vi "If Else X.vi"(0 "denge degeri":dbl, 5 "Xk":dbl, 7 "X(k-1)":dbl=0.1, 9 "output x 1":dbl, 11 "output x 2":dbl, 12 "result output x":dbl) -> (4 "Output X(k-1)":dbl format="%.4p", 15 "Start X":bool)   [LabVIEW 2014]
uses:
  Sub_VI/show_sensitivity.vi
  Sub_VI/global get findinput.vi
panel:
  out "cycle":bool
  in  "GPIB In":refnum<visa-resource-name>="GPIB0::8::INSTR"
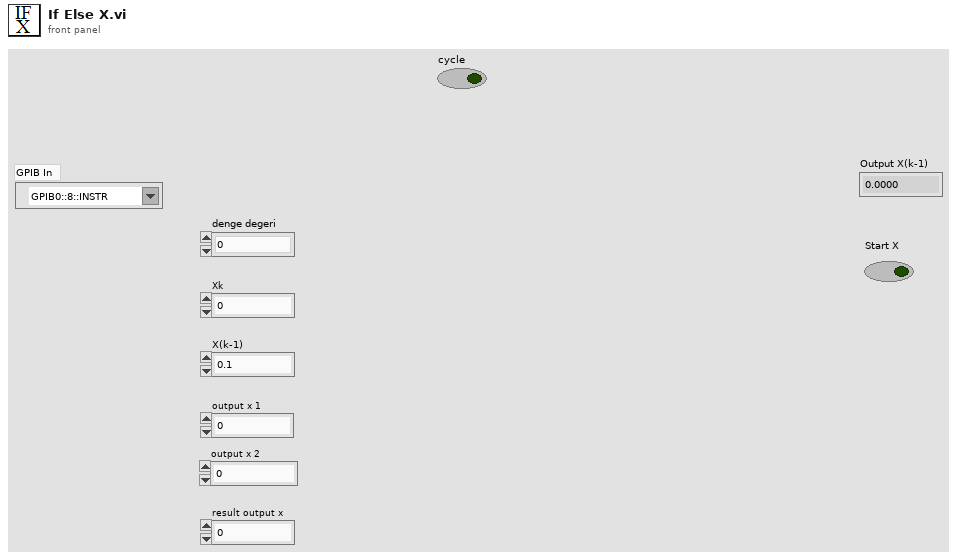
[diagram p1: front panel]
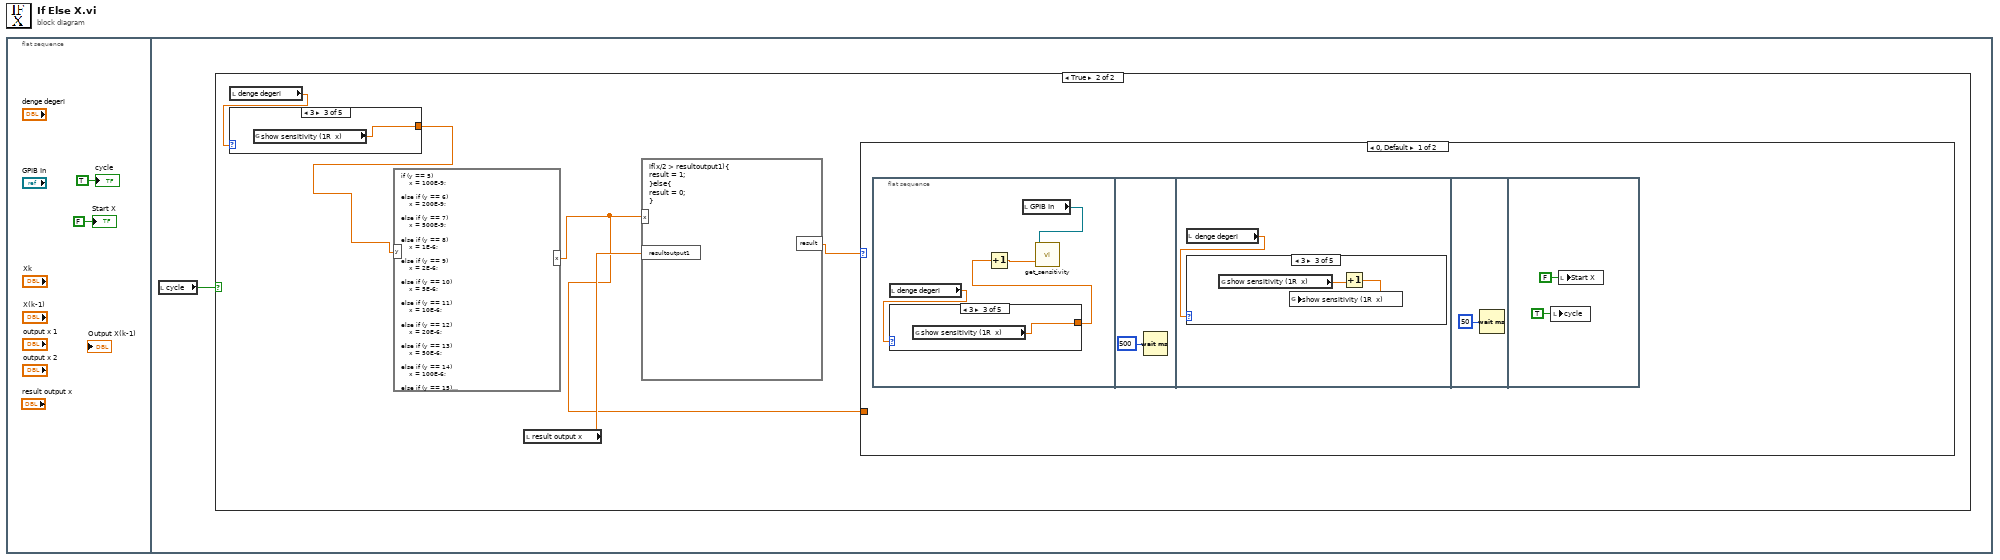
[diagram p0: block diagram]
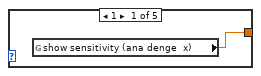
[diagram p3: hidden frame]
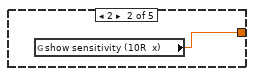
[diagram p4: hidden frame]
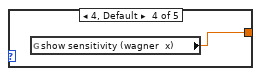
[diagram p5: hidden frame]
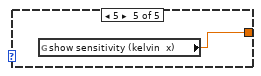
[diagram p6: hidden frame]
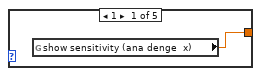
[diagram p7: hidden frame]
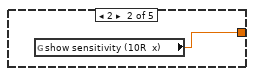
[diagram p8: hidden frame]
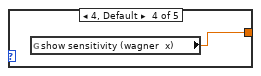
[diagram p9: hidden frame]
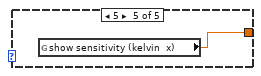
[diagram p10: hidden frame]
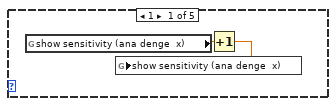
[diagram p11: hidden frame]
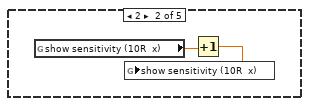
[diagram p12: hidden frame]
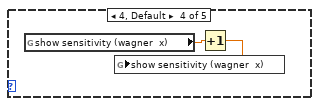
[diagram p13: hidden frame]
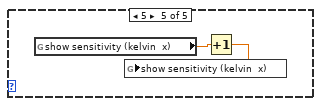
[diagram p14: hidden frame]
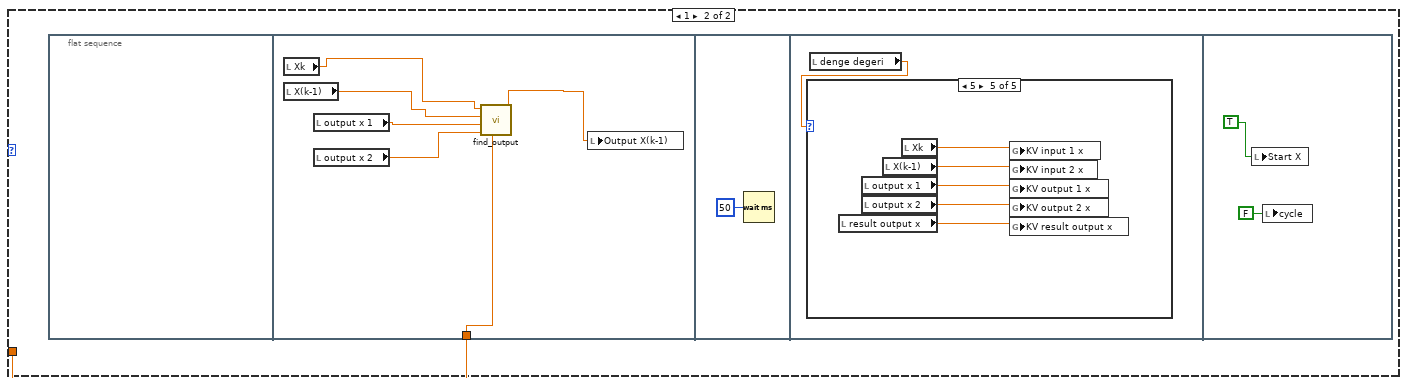
[diagram p15: hidden frame]
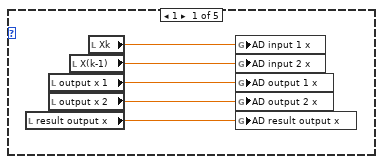
[diagram p16: hidden frame]
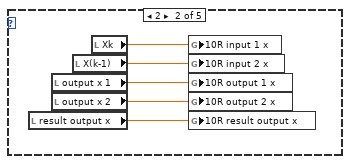
[diagram p17: hidden frame]
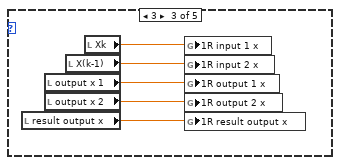
[diagram p18: hidden frame]
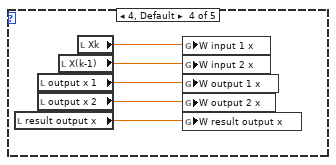
[diagram p19: hidden frame]
diagram:
  n1 = flat-sequence {
    frame #0 {
      "Start X" <- FALSE ("Start X")
      "cycle" <- TRUE ("Boolean")
    }
    frame #1 {
      n2 = local read "cycle"() -> (w3:bool)
      n3 = case shown="True" w3 {
        frame False {
        }
        frame True {
          n4 = local read "denge degeri"() -> (w5:dbl)
          n5 = case shown="3" w5 {
            tunnel: [w9 w10 w11 w12 w13] -> w4
            frame 1 {
              n6 = global read "show_sensitivity.vi" "show sensitivity (ana denge  x)"() -> (w9:dbl)
            }
            frame 2 {
              n7 = global read "show_sensitivity.vi" "show sensitivity (10R  x)"() -> (w10:dbl)
            }
            frame 3 {
              n8 = global read "show_sensitivity.vi" "show sensitivity (1R  x)"() -> (w11:dbl)
            }
            frame 4, Default {
              n9 = global read "show_sensitivity.vi" "show sensitivity (wagner  x)"() -> (w12:dbl)
            }
            frame 5 {
              n10 = global read "show_sensitivity.vi" "show sensitivity (kelvin  x)"() -> (w13:dbl)
            }
          }
          n11 = formula code="if (y == 5) \n    x = 100E-9;\n\nelse if (y == 6) \n    x = 200E-9;\n\nelse if (y == 7) \n    x = 500E-9;\n\nelse if (y == 8) \n    x = 1E-6;\n\nelse if (y == 9) \n    x = 2E-6;\n\nelse if (y == 10) \n    x = 5E-6;\n\nelse if (y == 11) \n    x = 10E-6;\n\nelse if (y == 12) \n    x = 20E-6;\n\nelse if (y == 13) \n    x = 50E-6;\n\nelse if (y == 14) \n    x = 100E-6;\n\nelse if (y == 15) \n    x = 200E-6;\n\nelse if (y == 16) \n    x = 500E-6;\n\nelse if (y == 17) \n    x = 1E-3;\n\nelse if (y == 18) \n    x = 2E-3;\n\nelse if (y == 19) \n    x = 5E-3;\n\nelse if (y == 20) \n    x = 10E-3;\n\nelse if (y == 21) \n    x = 20E-3;\n\nelse if (y == 22) \n    x = 50E-3;\n\nelse if (y == 23) \n    x = 100E-3;\n\nelse if (y == 24) \n    x = 200E-3;\n\nelse if (y == 25) \n    x = 500E-3;\n\nelse if (y == 26) \n    x = 1;\n\nelse \n    x = 1;"("y"=w4) -> ("x"=w6:dbl)
          n12 = local read "result output x"() -> (w8:dbl)
          n13 = formula code="if(x/2 > resultoutput1){\nresult = 1;\n}else{\nresult = 0;\n}"("x"=w6, "resultoutput1"=w8) -> ("result"=w7:dbl)
          n14 = case shown="0, Default" w7 {
            tunnel: w6 -> [_ w38]
            frame 0, Default {
              n15 = flat-sequence {
                frame #0 {
                  n16 = local read "denge degeri"() -> (w15:dbl)
                  n17 = case shown="3" w15 {
                    tunnel: [w18 w19 w20 w21 w22] -> w14
                    frame 1 {
                      n18 = global read "show_sensitivity.vi" "show sensitivity (ana denge  x)"() -> (w18:dbl)
                    }
                    frame 2 {
                      n19 = global read "show_sensitivity.vi" "show sensitivity (10R  x)"() -> (w19:dbl)
                    }
                    frame 3 {
                      n20 = global read "show_sensitivity.vi" "show sensitivity (1R  x)"() -> (w20:dbl)
                    }
                    frame 4, Default {
                      n21 = global read "show_sensitivity.vi" "show sensitivity (wagner  x)"() -> (w21:dbl)
                    }
                    frame 5 {
                      n22 = global read "show_sensitivity.vi" "show sensitivity (kelvin  x)"() -> (w22:dbl)
                    }
                  }
                  n23 = Increment(x=w14) -> (x+1=w16:dbl)
                  n24 = local read "GPIB In"() -> (w17:refnum<visa-resource-name>)
                  n25 = call "get_sensitivity.vi"("input 1"=w16, "SR850 GPIB In"=w17) -> ()  [unwired: 8 in, 2 out]
                }
                frame #1 {
                  n26 = Wait (ms)(milliseconds to wait=u32 500) -> ()  [unwired: 1 out]
                }
                frame #2 {
                  n27 = local read "denge degeri"() -> (w24:dbl)
                  n28 = case shown="3" w24 {
                    frame 1 {
                      n29 = global read "show_sensitivity.vi" "show sensitivity (ana denge  x)"() -> (w26:dbl)
                      n30 = Increment(x=w26) -> (x+1=w25:dbl)
                      n31 = global write "show_sensitivity.vi" "show sensitivity (ana denge  x)"(w25) -> ()
                    }
                    frame 2 {
                      n32 = global read "show_sensitivity.vi" "show sensitivity (10R  x)"() -> (w28:dbl)
                      n33 = Increment(x=w28) -> (x+1=w27:dbl)
                      n34 = global write "show_sensitivity.vi" "show sensitivity (10R  x)"(w27) -> ()
                    }
                    frame 3 {
                      n35 = global read "show_sensitivity.vi" "show sensitivity (1R  x)"() -> (w30:dbl)
                      n36 = Increment(x=w30) -> (x+1=w29:dbl)
                      n37 = global write "show_sensitivity.vi" "show sensitivity (1R  x)"(w29) -> ()
                    }
                    frame 4, Default {
                      n38 = global read "show_sensitivity.vi" "show sensitivity (wagner  x)"() -> (w32:dbl)
                      n39 = Increment(x=w32) -> (x+1=w31:dbl)
                      n40 = global write "show_sensitivity.vi" "show sensitivity (wagner  x)"(w31) -> ()
                    }
                    frame 5 {
                      n41 = global read "show_sensitivity.vi" "show sensitivity (kelvin  x)"() -> (w34:dbl)
                      n42 = Increment(x=w34) -> (x+1=w33:dbl)
                      n43 = global write "show_sensitivity.vi" "show sensitivity (kelvin  x)"(w33) -> ()
                    }
                  }
                }
                frame #3 {
                  n44 = Wait (ms)(milliseconds to wait=u32 50) -> ()  [unwired: 1 out]
                }
                frame #4 {
                  n45 = local write "cycle"(TRUE ("cycle")) -> ()
                  n46 = local write "Start X"(FALSE ("Start X")) -> ()
                }
              }
            }
            frame 1 {
              n47 = flat-sequence {
                tunnel: w38 -> [w42]
                frame #0 {
                }
                frame #1 {
                  n48 = local read "Xk"() -> (w41:dbl)
                  n49 = local read "X(k-1)"() -> (w40:dbl)
                  n50 = local read "output x 1"() -> (w44:dbl)
                  n51 = local read "output x 2"() -> (w43:dbl)
                  n52 = call "find_output.vi"("find output"=w42, "output 2"=w43, "output 1"=w44, "input 2"=w40, "input 1"=w41) -> ("getInput"=w39:dbl)  [unwired: 6 in]
                  n53 = local write "Output X(k-1)"(w39) -> ()
                }
                frame #2 {
                  n54 = Wait (ms)(milliseconds to wait=u32 50) -> ()  [unwired: 1 out]
                }
                frame #3 {
                  n55 = local read "denge degeri"() -> (w46:dbl)
                  n56 = case shown="5" w46 {
                    frame 1 {
                      n57 = local read "result output x"() -> (w47:dbl)
                      n58 = local read "output x 1"() -> (w49:dbl)
                      n59 = local read "output x 2"() -> (w48:dbl)
                      n60 = local read "X(k-1)"() -> (w50:dbl)
                      n61 = local read "Xk"() -> (w51:dbl)
                      n62 = global write "global get findinput.vi" "AD input 1 x"(w51) -> ()
                      n63 = global write "global get findinput.vi" "AD input 2 x"(w50) -> ()
                      n64 = global write "global get findinput.vi" "AD output 1 x"(w49) -> ()
                      n65 = global write "global get findinput.vi" "AD output 2 x"(w48) -> ()
                      n66 = global write "global get findinput.vi" "AD result output x"(w47) -> ()
                    }
                    frame 2 {
                      n67 = local read "result output x"() -> (w56:dbl)
                      n68 = local read "output x 1"() -> (w54:dbl)
                      n69 = local read "output x 2"() -> (w55:dbl)
                      n70 = local read "X(k-1)"() -> (w53:dbl)
                      n71 = local read "Xk"() -> (w52:dbl)
                      n72 = global write "global get findinput.vi" "10R input 1 x"(w52) -> ()
                      n73 = global write "global get findinput.vi" "10R input 2 x"(w53) -> ()
                      n74 = global write "global get findinput.vi" "10R output 1 x"(w54) -> ()
                      n75 = global write "global get findinput.vi" "10R output 2 x"(w55) -> ()
                      n76 = global write "global get findinput.vi" "10R result output x"(w56) -> ()
                    }
                    frame 3 {
                      n77 = local read "result output x"() -> (w61:dbl)
                      n78 = local read "output x 1"() -> (w59:dbl)
                      n79 = local read "output x 2"() -> (w60:dbl)
                      n80 = local read "X(k-1)"() -> (w58:dbl)
                      n81 = local read "Xk"() -> (w57:dbl)
                      n82 = global write "global get findinput.vi" "1R input 1 x"(w57) -> ()
                      n83 = global write "global get findinput.vi" "1R input 2 x"(w58) -> ()
                      n84 = global write "global get findinput.vi" "1R output 1 x"(w59) -> ()
                      n85 = global write "global get findinput.vi" "1R output 2 x"(w60) -> ()
                      n86 = global write "global get findinput.vi" "1R result output x"(w61) -> ()
                    }
                    frame 4, Default {
                      n87 = local read "result output x"() -> (w66:dbl)
                      n88 = local read "output x 1"() -> (w64:dbl)
                      n89 = local read "output x 2"() -> (w65:dbl)
                      n90 = local read "X(k-1)"() -> (w63:dbl)
                      n91 = local read "Xk"() -> (w62:dbl)
                      n92 = global write "global get findinput.vi" "W input 1 x"(w62) -> ()
                      n93 = global write "global get findinput.vi" "W input 2 x"(w63) -> ()
                      n94 = global write "global get findinput.vi" "W output 1 x"(w64) -> ()
                      n95 = global write "global get findinput.vi" "W output 2 x"(w65) -> ()
                      n96 = global write "global get findinput.vi" "W result output x"(w66) -> ()
                    }
                    frame 5 {
                      n97 = local read "result output x"() -> (w71:dbl)
                      n98 = local read "output x 1"() -> (w69:dbl)
                      n99 = local read "output x 2"() -> (w70:dbl)
                      n100 = local read "X(k-1)"() -> (w68:dbl)
                      n101 = local read "Xk"() -> (w67:dbl)
                      n102 = global write "global get findinput.vi" "KV input 1 x"(w67) -> ()
                      n103 = global write "global get findinput.vi" "KV input 2 x"(w68) -> ()
                      n104 = global write "global get findinput.vi" "KV output 1 x"(w69) -> ()
                      n105 = global write "global get findinput.vi" "KV output 2 x"(w70) -> ()
                      n106 = global write "global get findinput.vi" "KV result output x"(w71) -> ()
                    }
                  }
                }
                frame #4 {
                  n107 = local write "Start X"(TRUE ("START X")) -> ()
                  n108 = local write "cycle"(FALSE ("cycle")) -> ()
                }
              }
            }
          }
        }
      }
    }
  }
